vi "Initialize Hardware References.vi"(8 "error in (no error)":errorcluster caption="错误输入（无错误）", 11 "Hardware Resources in":T1={"电压读取设置"={"DAQmx Channel"="", "Max Input"=0.0, "Min Input"=0.0, "Sample Rate"=0.0, "Sample Number"=0, "DAQmx Task"="", "device in"=""}, "角度传感器设置"={"counter"="Dev1/ctr0", "units"=10146, "分辨率"=0, "初始角度"=0.0, "DecodingType"=10092, "A相端口"="/Dev1/PFI8", "B相端口"="/Dev1/PFI8", "task in"=""}} caption="硬件资源输入" {"角度传感器设置"."DecodingType" items=["X1"=10090, "X2"=10091, "X4"=10092, "Two Pulse Counting"=10313]; "角度传感器设置"."units" items=["Degrees"=10146, "Radians"=10273, "Ticks"=10304, "From Custom Scale"=10065]}) -> (0 "error out":errorcluster caption="错误输出", 3 "Hardware Resources out":T1={"电压读取设置"={"DAQmx Channel"="", "Max Input"=0.0, "Min Input"=0.0, "Sample Rate"=0.0, "Sample Number"=0, "DAQmx Task"="", "device in"=""}, "角度传感器设置"={"counter"="Dev1/ctr0", "units"=10146, "分辨率"=0, "初始角度"=0.0, "DecodingType"=10092, "A相端口"="/Dev1/PFI8", "B相端口"="/Dev1/PFI8", "task in"=""}} caption="硬件资源输出" {"角度传感器设置"."DecodingType" items=["X1"=10090, "X2"=10091, "X4"=10092, "Two Pulse Counting"=10313]; "角度传感器设置"."units" items=["Degrees"=10146, "Radians"=10273, "Ticks"=10304, "From Custom Scale"=10065]})   [LabVIEW 2015, in "Acquisition.lvlib"]
doc: "初始化硬件引用。"
uses:
  Acquisition.lvlib
  Hardware Configuration.ctl
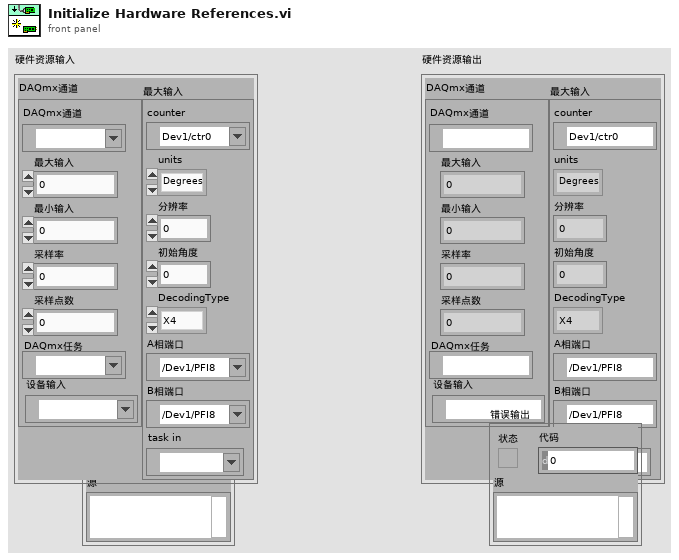
[diagram p1: front panel]
types:
  T1 = typedef "Acquisition.lvlib/Hardware Configuration.ctl" = cluster{"电压读取设置":cluster{"DAQmx Channel":tag, "Max Input":dbl, "Min Input":dbl, "Sample Rate":dbl, "Sample Number":i32, "DAQmx Task":refnum<k21>, "device in":tag}, "角度传感器设置":cluster{"counter":tag, "units":i32, "分辨率":i32, "初始角度":dbl, "DecodingType":i32, "A相端口":tag, "B相端口":tag, "task in":refnum<k21>}}
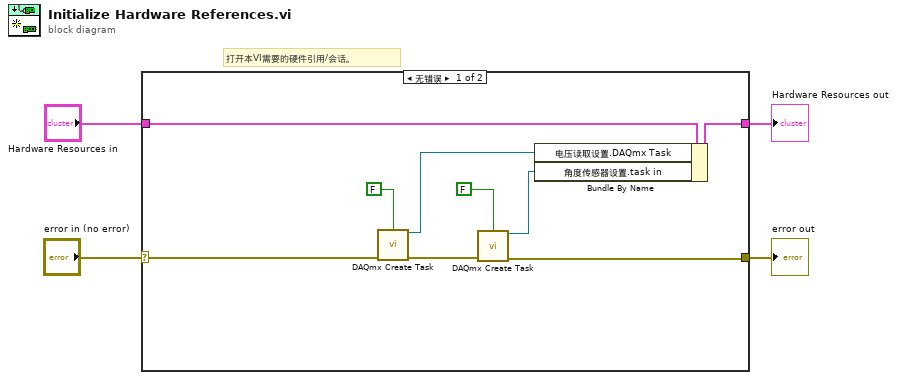
[diagram p0: block diagram]
diagram:
  # "打开本VI需要的硬件引用/会话。"
  n1 = case shown="无错误" "error in (no error)" {
    selector: "error in (no error)" -> [w5 w14]
    tunnel: [w8 w14] -> w3
    tunnel: "Hardware Resources in" -> [w6 w15]
    tunnel: [w13 w15] -> w1
    frame No Error {
      n2 = call <vilib>:"DAQmx Create Task.vi"("auto cleanup"=FALSE, "error in"=w5) -> ("task out"=w11:refnum<k21>, "error out"=w9:errorcluster)  [unwired: 12 in]
      n3 = call <vilib>:"DAQmx Create Task.vi"("auto cleanup"=FALSE, "error in"=w9) -> ("task out"=w7:refnum<k21>, "error out"=w8:errorcluster)  [unwired: 12 in]
      n4 = Bundle By Name(cluster=w6, "电压读取设置.DAQmx Task"=w11, "角度传感器设置.task in"=w7) -> (w13:T1)
    }
    frame Error {
    }
  }
  "Hardware Resources out" <- w1
  "error out" <- w3
